vi "Lezeti_Power_Monitor_05.vi"() -> ()   [LabVIEW 2012]
doc: "This example shows how to use autosetup and acquire a waveform on a single channel."
uses:
  <instrlib>/RIGOL DS1000 Series/Public/Data/Read (Single Waveform).vi
  <vilib>/measure/madcrms.llb/Basic Averaged DC-RMS for 1 Chan.vi
  <vilib>/measure/mascope.llb/Cycle Average and RMS 1 chan.vi
  <vilib>/Utility/file.llb/Write To Spreadsheet File (DBL).vi
  <instrlib>/RIGOL DS1000 Series/RIGOL DS1000 Series.lvlib
  <vilib>/measure/NI_MAPro.lvlib
panel:
  out "Elapsed Time (s)":dbl
  in  "Output File":path
  out "Average Power (Watts)":dbl
  out "Instant Power Waveform":waveform(dbl)(graph)
  in  "Current Channel":u16(ring) items=["Channel 1", "Channel 2", "Channel 3", "Channel 4"]
  in  "Timeout":u32=10000
  out "IRMS":dbl
  out "Current Waveform":waveform(dbl)(graph)
  out "VRMS":dbl
  in  "Voltage Channel":u16(ring) items=["Channel 1", "Channel 2", "Channel 3", "Channel 4"]
  in  "Stop":bool
  in  "Timeout":u32=10000
  out "Voltage Waveform":waveform(dbl)(graph)
  in  "VISA resource name":refnum<visa-resource-name>
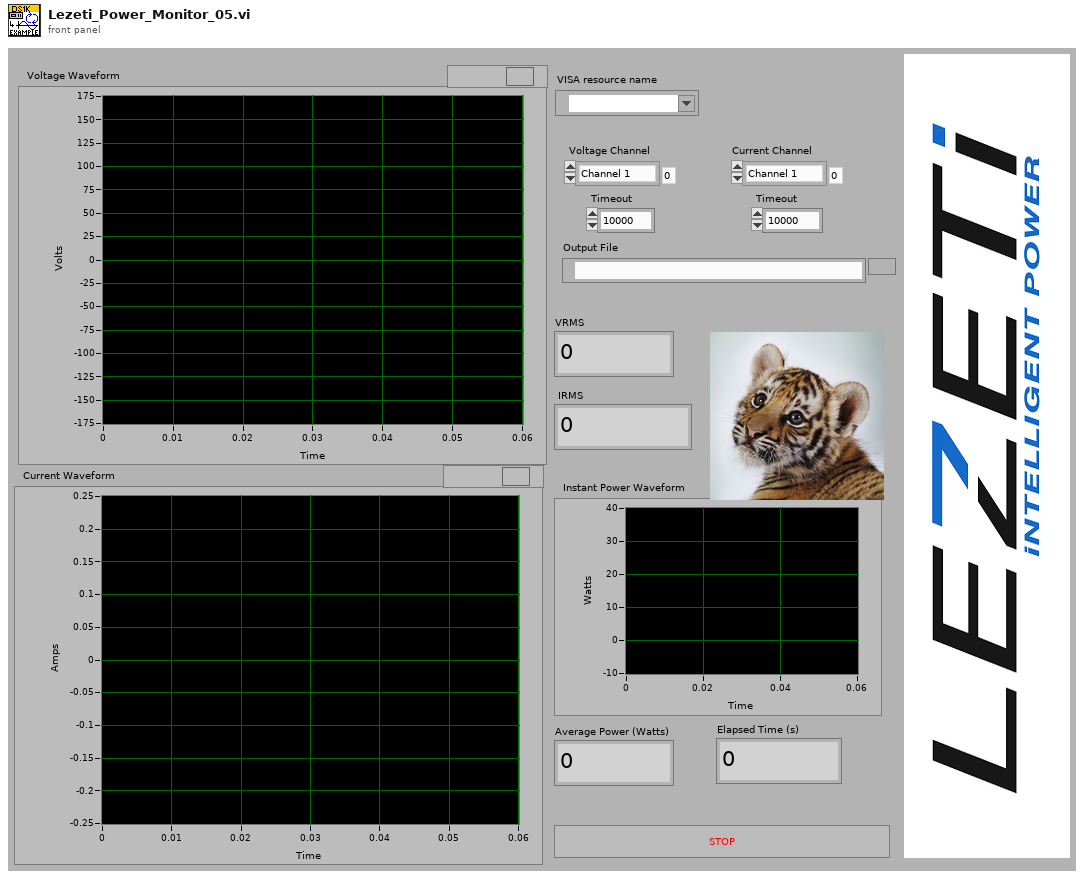
[diagram p1: front panel]
types:
  T1 = typedef "NI_Matrix.lvlib/RealMatrix.ctl" = dbl[][]
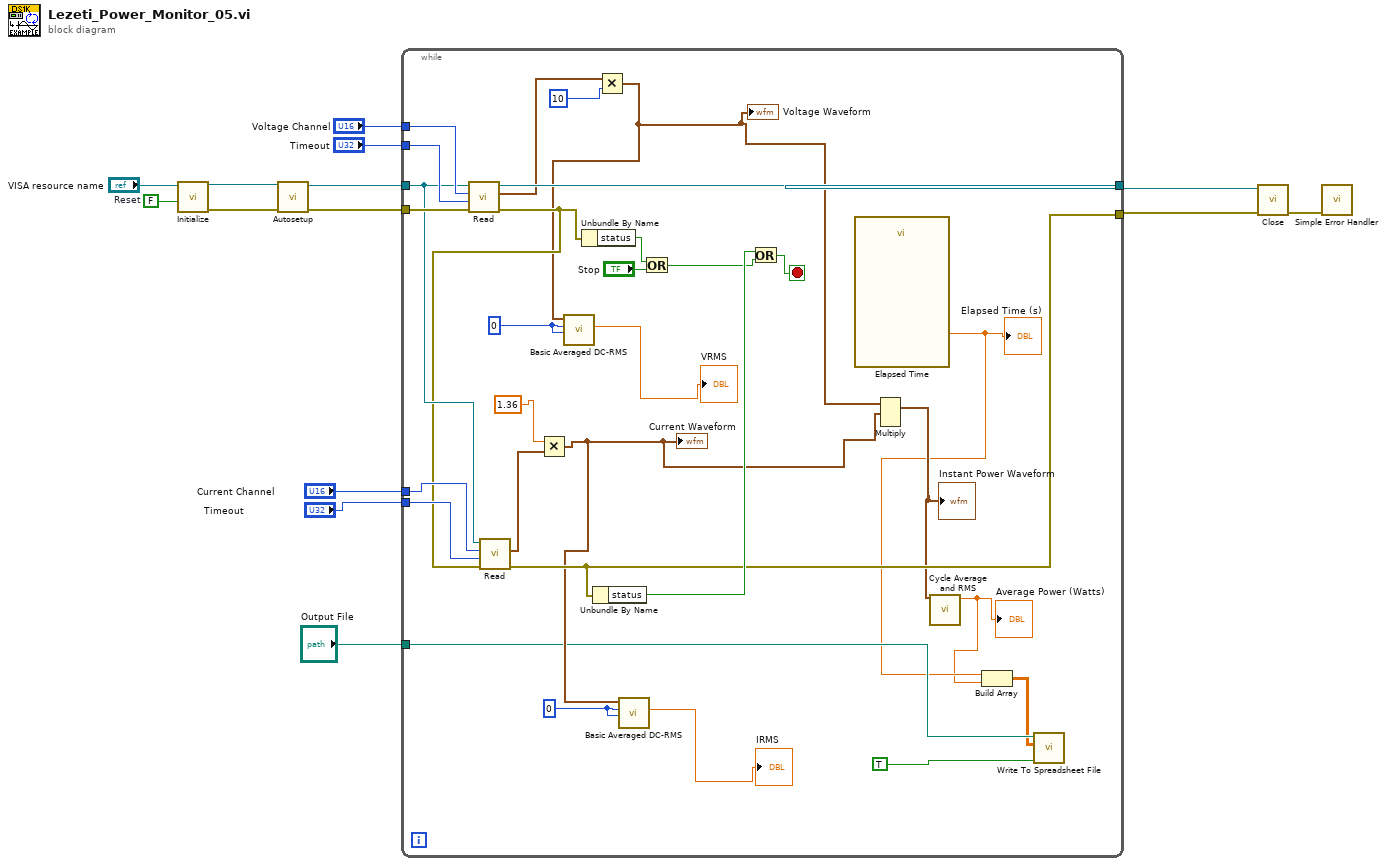
[diagram p0: block diagram]
diagram:
  w5 = FALSE  # Reset
  n1 = call <instrlib>:"Initialize.vi"("Reset (True)"=w5, "VISA resource name"="VISA resource name") -> ("error out"=w10:errorcluster, "VISA resource name out"=w9:refnum<visa-resource-name>)  [unwired: 2 in, 6 out]
  n2 = call <instrlib>:"Autosetup.vi"("error in (no error)"=w10, "VISA resource name"=w9) -> ("error out"=w7:errorcluster, "VISA resource name out"=w8:refnum<visa-resource-name>)  [unwired: 8 out]
  n3 = while {
    tunnel: w8 -> [w33]
    tunnel: w7 -> [w44]
    tunnel: [w43] -> w13
    tunnel: "Timeout" -> [w39]
    tunnel: "Voltage Channel" -> [w40]
    tunnel: "Current Channel" -> [w35]
    tunnel: "Timeout" -> [w34]
    tunnel: [w31] -> w2
    tunnel: "Output File" -> [w19]
    stop <- w21 stop-if-true
    w36 = 0
    w38 = 0
    n4 = call-poly <instrlib>:"Read.vi"("error in (no error)"=w44, "Timeout (10000 ms)"=w39, "Channel (0: Channel 1)"=w40, "VISA resource name"=w33) -> ("error out"=w32:errorcluster, "Waveform Data"=w29:waveform(dbl), "VISA resource name out"=w43:refnum<visa-resource-name>)  [unwired: 5 out]
    n5 = call-poly <instrlib>:"Read.vi"("error in (no error)"=w32, "Timeout (10000 ms)"=w34, "Channel (0: Channel 1)"=w35, "VISA resource name"=w33) -> ("error out"=w31:errorcluster, "Waveform Data"=w26:waveform(dbl))  [unwired: 6 out]
    n6 = Multiply(x=1.36, y=w26) -> (x*y=w23:waveform(dbl))
    "Current Waveform" <- w23
    n7 = Unbundle By Name(w32) -> ("status"=w42:bool)
    n8 = Unbundle By Name(w31) -> ("status"=w37:bool)
    n9 = Multiply(x=w29, y=10) -> (x*y=w28:waveform(dbl))
    "Voltage Waveform" <- w28
    n10 = call-poly <vilib>:"Basic Averaged DC-RMS.vi"("window"=w38, "averaging type"=w38, "signal in"=w28) -> ("RMS value"=→"VRMS":dbl)  [unwired: 5 in, 3 out]
    n11 = call-poly <vilib>:"Basic Averaged DC-RMS.vi"("window"=w36, "averaging type"=w36, "signal in"=w23) -> ("RMS value"=→"IRMS":dbl)  [unwired: 5 in, 3 out]
    n12 = Or(x=w42, y="Stop") -> (x .or. y?=w22:bool)
    n13 = Or(x=w37, y=w22) -> (x .or. y?=w21:bool)
    n14 = call "Elapsed Time"() -> ("Elapsed Time (s)"=w17:dbl)  [unwired: 12 in, 7 out]
    "Elapsed Time (s)" <- w17
    n15 = Multiply(1:w23, 2:w28) -> (0:w20:waveform(dbl))  [unwired: 1 in, 1 out]
    "Instant Power Waveform" <- w20
    n16 = call-poly <vilib>:"Cycle Average and RMS.vi"("signal in"=w20) -> ("cycle average"=w16:dbl)  [unwired: 7 in, 3 out]
    "Average Power (Watts)" <- w16
    n17 = Build Array(w17, w16) -> (w15:T1)
    n18 = call-poly <vilib>:"Write To Spreadsheet File.vi"("append to file? (new file:F)"=TRUE, "2D data"=w15, "file path (dialog if empty)"=w19) -> ()  [unwired: 5 in, 1 out]
  }
  n19 = call <instrlib>:"Close.vi"("error in (no error)"=w2, "VISA resource name"=w13) -> ("error out"=w14:errorcluster)  [unwired: 9 out]
  n20 = call <vilib>:"Simple Error Handler.vi"("error in (no error)"=w14) -> ()  [unwired: 1 in, 8 out]
